vi "Encoder Position & Velocity (FPGA).vi"(5 "Position Reset":bool) -> (2 "Position (Counts)":i32)   [LabVIEW 2013]
doc: "This is an FPGA vi for Quadrature Encoder Velocity and Acceleration Estimation using CompactRIO. It requires as inputs a Fixed Time Interval for velocity and acceleration estimation.\n\nThis application is designed to work with an R-Series expansion setup using PCI/PXI-7811R FPGA device and a CompactRIO cRIO-9411 digital input module installed in slot 1 of the expansion chassis."
uses:
  <vilib>/eio/EIONode/EIONode.xnode
  <vilib>/rvi/Arithmetic/AddSubMult/XNode/nirviSatArithmetic.xnode
  <vilib>/rvi/eio/common/nirviEmuTemplateMethod_errors.vi
  <instrlib>/_niInstr/Basic Elements/v1/FPGA/niInstr Basic Elements v1 FPGA.lvlib
  <instrlib>/_niInstr/Basic Elements/v1/FPGA/Private/Count Up U64.vi
panel:
  out "count out 4":u64
  out "count out 3":u64
  out "Mod1/DI2":bool
  out "Mod1/DI1":bool
  out "Mod1/DI0":bool
  out "count out 2":i32
  out "count out 1":i32
  in  "stop":bool
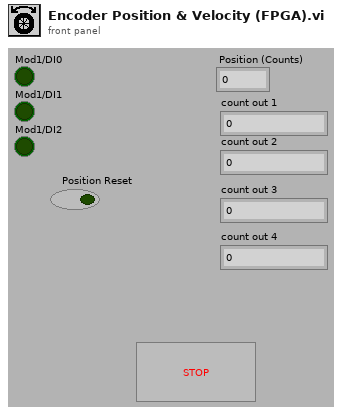
[diagram p1: front panel]
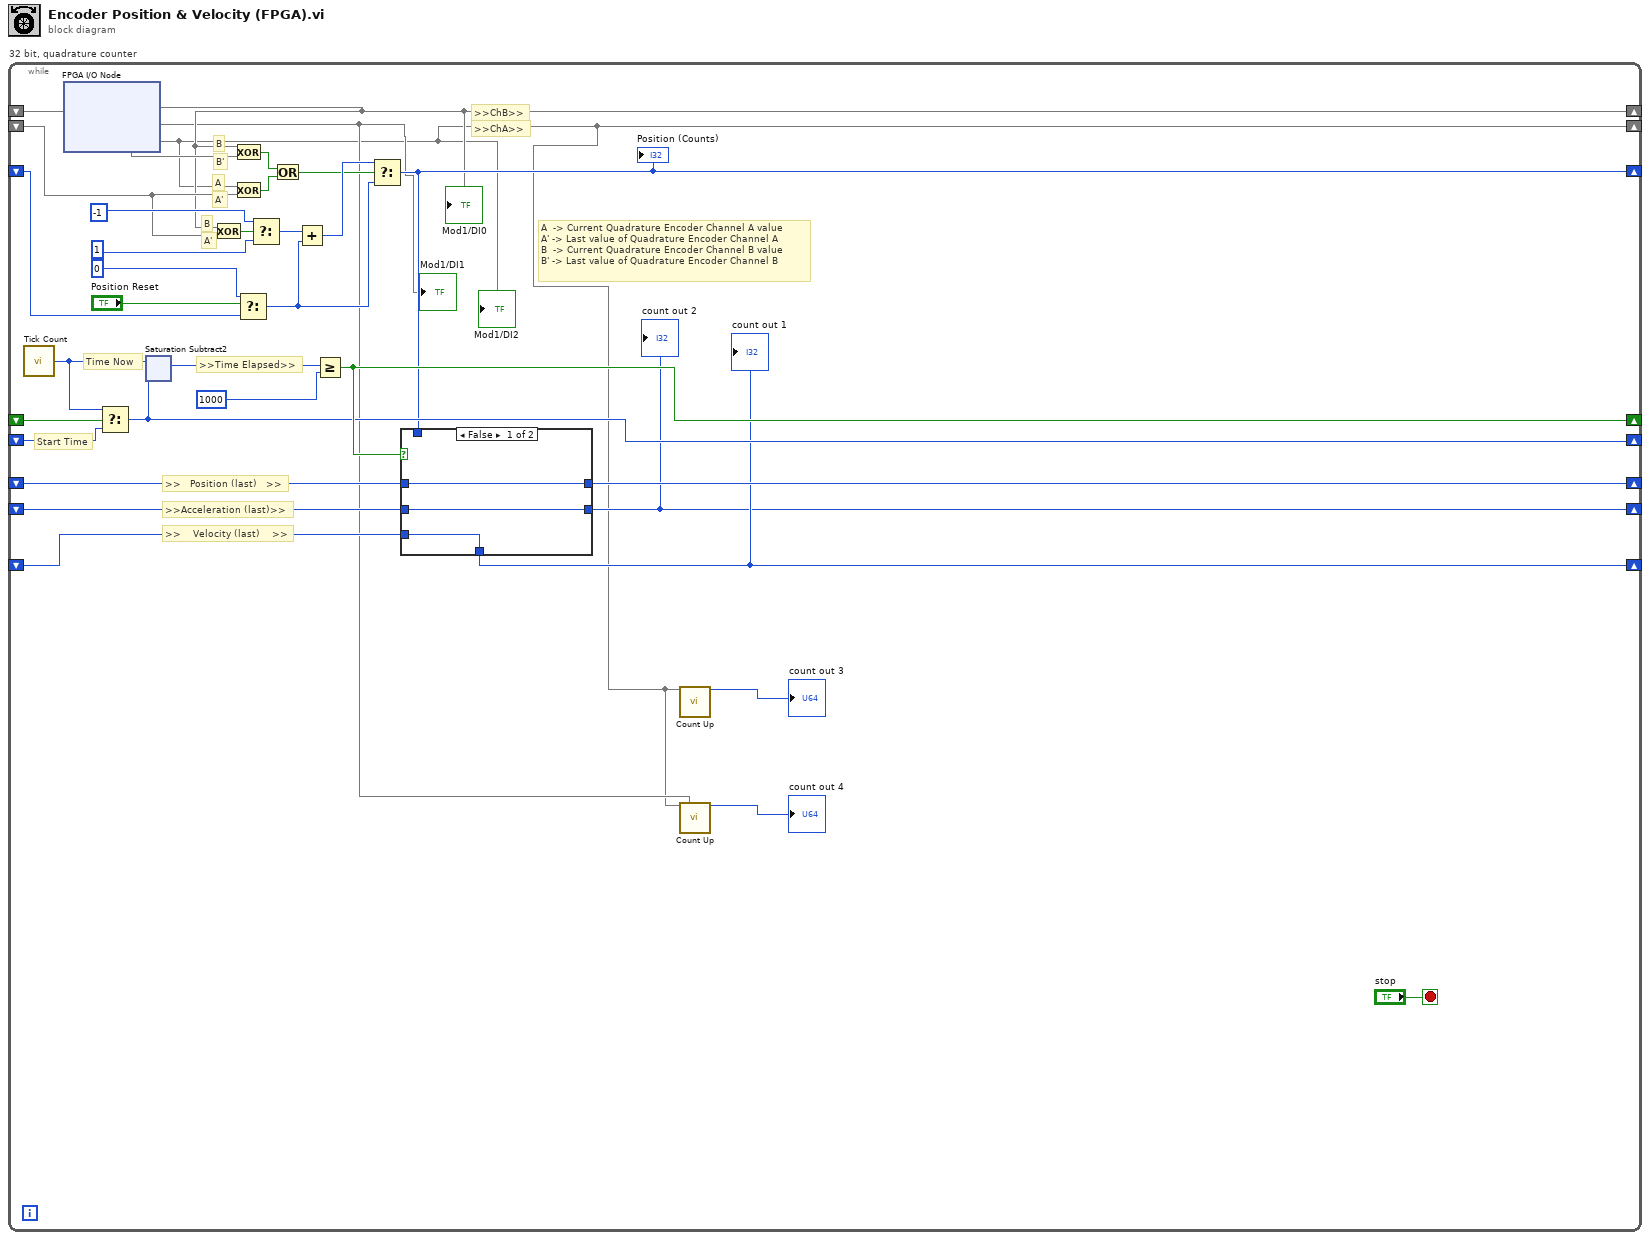
[diagram p0: block diagram]
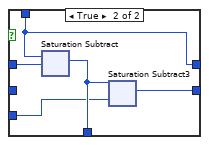
[diagram p2: hidden frame]
diagram:
  n1 = while "32 bit, quadrature counter" {
    shift-right: [w5] -> _
    shift-left: _ -> [w10]
    shift-right: [w9] -> _
    shift-left: _ -> [w21]
    shift-right: [w1] -> _
    shift-left: _ -> [w24]
    shift-right: [w17] -> _
    shift-left: _ -> [w20]
    shift-right: [w12] -> _
    shift-left: _ -> [w18]
    shift-right: [w8] -> _
    shift-left: _ -> [w15]
    shift-right: [w7] -> _
    shift-left: _ -> [w14]
    shift-right: [w6] -> _
    shift-left: _ -> [w11]
    stop <- "stop" stop-if-true
    # "A  -> Current Quadrature Encoder Channel A value\nA' -> Last value of Quadrature Encoder Channel A\nB  -> Current Quadrature Encoder Channel B value\nB' -> Last value of Quadrature Encoder Channel B"
    # ">>Acceleration (last)>>"
    # "Start Time"
    # "A'"
    # "B"
    # "A'"
    # "A"
    # "B'"
    # "B"
    # ">>ChB>>"
    # ">>ChA>>"
    # ">>    Velocity (last)    >>"
    # ">>   Position (last)   >>"
    # "Time Now"
    # ">>Time Elapsed>>"
    n2 = call "Tick Count"() -> ("Tick Count(uSec)"=w13:u32)
    n3 = xnode "FPGA I/O Node"() -> ("Mod1/DI0"=w5, "Mod1/DI1"=w2, "Mod1/DI2"=w1)  [unwired: 3 in, 3 out]
    "Mod1/DI0" <- w5
    "Mod1/DI1" <- w2
    "Mod1/DI2" <- w1
    n4 = Select(t=w13, s=w20, f=w18) -> (s? t:f=w12:u32)
    n5 = xnode ("Saturation Subtract2")("x"=w13, "y"=w12) -> ("x-y"=w16:u32)
    n6 = Exclusive Or(1:w24, 2:w5) -> (0:w25:bool)
    n7 = Exclusive Or(1:w10, 2:w5) -> (0:w26:bool)
    n8 = Exclusive Or(1:w24, 2:w1) -> (0:w27:bool)
    n9 = Select(t=0 ("32 bit"), s="Position Reset", f=w21) -> (s? t:f=w32:i32)
    n10 = Select(t=-1 ("32 bit"), s=w25, f=1 ("32 bit")) -> (s? t:f=w30:i32)
    n11 = Or(x=w26, y=w27) -> (x .or. y?=w22:bool)
    n12 = Add(x=w30, y=w32) -> (x+y=w34:i32)
    n13 = Greater Or Equal?(x=w16, y=u32 1000 ("Velocity Interval (uSec)")) -> (x >= y?=w17:bool)
    n14 = Select(t=w34, s=w22, f=w32) -> (s? t:f=w9:i32)
    "Position (Counts)" <- w9
    n15 = case shown="False" w17 {
      tunnel: w9 -> [_ w48]
      tunnel: w15 -> [w45 w52]
      tunnel: [w47 w51] -> w7
      tunnel: w14 -> [w47 w50]
      tunnel: [w46 w49] -> w6
      tunnel: w11 -> [w46 _]
      tunnel: [w45 w48] -> w8
      frame False {
      }
      frame True {
        n16 = xnode ("Saturation Subtract")("x"=w48, "y"=w52) -> ("x-y"=w51:i32)
        n17 = xnode ("Saturation Subtract3")("x"=w51, "y"=w50) -> ("x-y"=w49:i32)
      }
    }
    "count out 1" <- w7
    "count out 2" <- w6
    n18 = call-poly <instrlib>:"Count Up.vi"("increment"=w1) -> ("count out"=→"count out 3":u64)  [unwired: 14 in]
    n19 = call-poly <instrlib>:"Count Up.vi"("increment"=w1, "reset"=w2) -> ("count out"=→"count out 4":u64)  [unwired: 13 in]
  }
